vi "Write Data.vi"(10 "Data":i32, 11 "Addition Task Msg in":refnum<class "Addition Task Msg.lvclass">) -> (3 "Addition Task Msg out":refnum<class "Addition Task Msg.lvclass">)   [LabVIEW 2015, in "Addition Actor.lvlib" / "Addition Task Msg.lvclass"]
uses:
  Addition Task Msg.lvclass
  Addition Task Msg.lvclass/Addition Task Msg.ctl
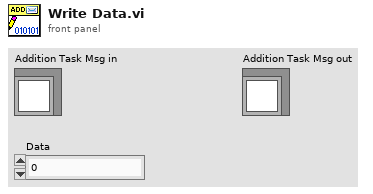
[diagram p1: front panel]
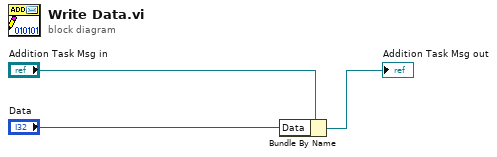
[diagram p0: block diagram]
diagram:
  n1 = Bundle By Name(cluster="Addition Task Msg in", "Data"="Data") -> (→"Addition Task Msg out":refnum<class "Addition Task Msg.lvclass">)
